vi "SEN_Loop.vi"() -> ()   [LabVIEW 2023, in "GameController_SEN.lvlib"]
uses:
  GameController_SEN.lvlib
  ENUM_SEN_State.ctl
  <vilib>/Rock Robotics/WPI/Joystick/WPI_JoystickDevRef.ctl
  <vilib>/Rock Robotics/WPI/Joystick/WPI_JoystickDeviceEnum.ctl
  ENUM_SEN_Action.ctl
  RoboRIO Utilities/Global_STOP.vi
  Global_SEN_Data Out.vi
panel:
  out "Input Bool Data":bool
  out "Output DBL Data":dbl
  out "Cycle Time (S)":dbl format="%.3g"
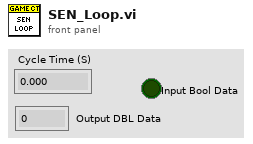
[diagram p1: front panel]
types:
  T1 = typedef "WPI_JoystickDevRef.ctl" = cluster{"Device":T2}
  T2 = typedef "WPI_JoystickDeviceEnum.ctl" = enum16{"USB 0", "USB 1", "USB 2", "USB 3", "USB 4", "USB 5"}
  T3 = typedef "GameController_SEN.lvlib/ENUM_SEN_State.ctl" = enum16{"Startup", "Enable", "Shutdown"}
  T4 = typedef "GameController_SEN.lvlib/ENUM_SEN_Action.ctl" = enum16{"No Action", "Reset Time", "Read Enable", "Read Disable"}
  T5 = cluster{"Sensor Ref 1":T1, "Sensor Ref 0":T1, "State":T3, "Previous State":T3, "Current Time":timestamp, "Previous Time":timestamp, "Start Time":timestamp, "Target Time (ms)":u32, "Cycle Time(S)":dbl, "SEN Input":bool, "SEN Output DBL":dbl, "Read Enable":bool, "Axes 0":dbl[], "Buttons 0":bool[], "POVs 0":i16[], "Axes 1":dbl[], "Buttons 1":bool[], "POVs 1":i16[]}
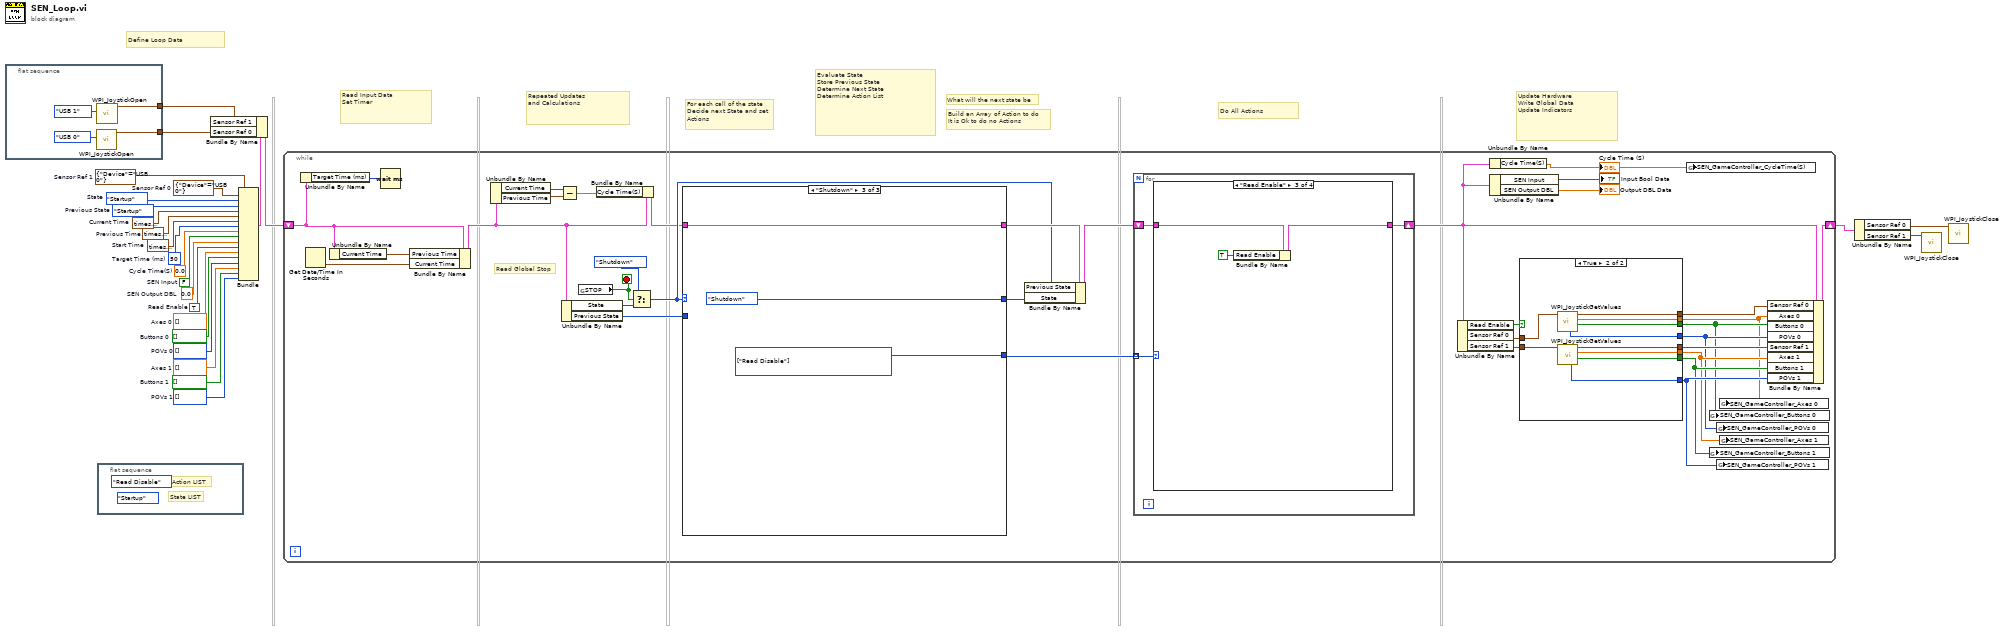
[diagram p0: block diagram]
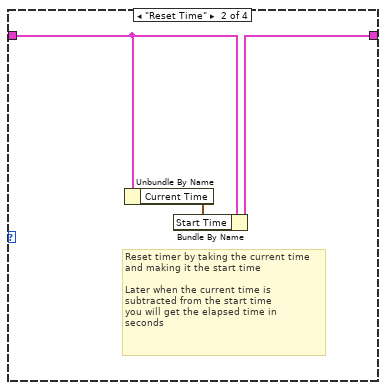
[diagram p4: hidden frame]
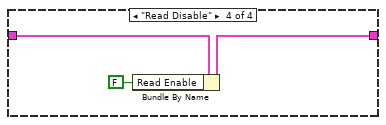
[diagram p5: hidden frame]
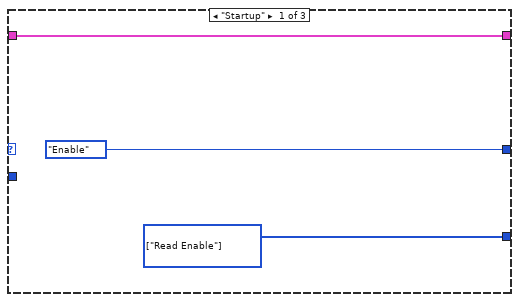
[diagram p6: hidden frame]
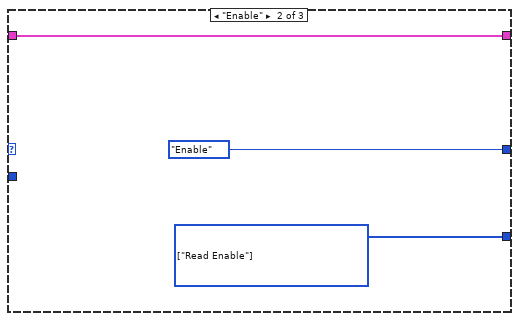
[diagram p7: hidden frame]
diagram:
  w1 = T1 {"Device"=enum."USB 0"}  # Sensor Ref 0
  w2 = T1 {"Device"=enum."USB 0"}  # Sensor Ref 1
  w5 = i16[] []  # POVs 1
  w6 = bool[] []  # Buttons 1
  w7 = dbl[] []  # Axes 1
  w8 = i16[] []  # POVs 0
  w9 = bool[] []  # Buttons 0
  w10 = dbl[] []  # Axes 0
  w15 = TRUE  # Read Enable
  w17 = 0.0  # Cycle Time(S)
  w18 = ENUM_SEN_State."Startup"  # Previous State
  w19 = timestamp(0 s since 1904-01-01)  # Previous Time
  w20 = u32 50  # Target Time (ms)
  w21 = 0.0  # SEN Output DBL
  w22 = FALSE  # SEN Input
  w23 = timestamp(0 s since 1904-01-01)  # Start Time
  w24 = timestamp(0 s since 1904-01-01)  # Current Time
  w25 = ENUM_SEN_State."Startup"  # State
  # "Build an Array of Action to do\nIt is Ok to do no Actions"
  # "What will the next state be"
  # "For each call of the state\nDecide next State and set\nActions"
  # "Define Loop Data"
  # "Repeated Updates\nand Calculations"
  # "Read Input Data\nSet Timer"
  # "Evaluate State\nStore Previous State\nDetermine Next State\nDetermine Action List"
  # "Do All Actions"
  # "Update Hardware\nWrite Global Data\nUpdate Indicators"
  n1 = flat-sequence {
    tunnel: [w28] -> w12
    tunnel: [w26] -> w11
    frame #0 {
      n2 = call <vilib>:"WPI_JoystickOpen.vi"("JoystickDevice"=WPI_JoystickDeviceEnum."USB 0") -> ("JoystickDevRef"=w28:T1)  [unwired: 10 in]
      n3 = call <vilib>:"WPI_JoystickOpen.vi"("JoystickDevice"=WPI_JoystickDeviceEnum."USB 1") -> ("JoystickDevRef"=w26:T1)  [unwired: 10 in]
    }
  }
  n4 = flat-sequence {
    frame #0 {
      (unwired) ENUM_SEN_State."Startup" ("State")
      (unwired) ENUM_SEN_Action."Read Disable" ("Action")
      # "State LIST"
      # "Action LIST"
    }
  }
  n5 = Bundle("Sensor Ref 1"=w2, "Sensor Ref 0"=w1, "State"=w25, "Previous State"=w18, "Current Time"=w24, "Previous Time"=w19, "Start Time"=w23, "Target Time (ms)"=w20, "Cycle Time(S)"=w17, "SEN Input"=w22, "SEN Output DBL"=w21, "Read Enable"=w15, "Axes 0"=w10, "Buttons 0"=w9, "POVs 0"=w8, "Axes 1"=w7, "Buttons 1"=w6, "POVs 1"=w5) -> (w14:T5)  [unwired: 1 in]
  n6 = Bundle By Name(cluster=w14, "Sensor Ref 1"=w11, "Sensor Ref 0"=w12) -> (w13:T5)
  n7 = while {
    shift-right: [w41] -> w16
    shift-left: w13 -> [w54]
    stop <- w59 stop-if-true
    # "Read Global Stop"
    n8 = Unbundle By Name(w54) -> ("Target Time (ms)"=w56:u32)
    n9 = Get Date/Time In Seconds() -> (seconds since 1Jan1904=w63:timestamp)
    n10 = Unbundle By Name(w54) -> ("Current Time"=w55:timestamp)
    n11 = Wait (ms)(milliseconds to wait=w56) -> ()  [unwired: 1 out]
    n12 = Bundle By Name(cluster=w54, "Previous Time"=w55, "Current Time"=w63) -> (w48:T5)
    n13 = Unbundle By Name(w48) -> ("Current Time"=w49:timestamp, "Previous Time"=w50:timestamp)
    n14 = Subtract(x=w49, y=w50) -> (x-y=w46:dbl)
    n15 = Unbundle By Name(w48) -> ("State"=w57:T3, "Previous State"=w53:T3)
    n16 = global read "Global_STOP.vi" "STOP"() -> (w59:bool)
    n17 = Bundle By Name(cluster=w48, "Cycle Time(S)"=w46) -> (w47:T5)
    n18 = Select(t=ENUM_SEN_State."Shutdown" ("State"), s=w59, f=w57) -> (s? t:f=w51:T3)
    n19 = case shown="\"Shutdown\"" w51 {
      tunnel: w47 -> [w91 w92 w97]
      tunnel: [w91 w92 w97] -> w61
      tunnel: [ENUM_SEN_State."Enable" ("State") ENUM_SEN_State."Enable" ("State") ENUM_SEN_State."Shutdown" ("State")] -> w60
      tunnel: [w90 w94 w95] -> w45
      tunnel: w53 -> [_ _ _]
      frame "Startup" {
        w90 = T4[] [enum."Read Enable"] items=["No Action", "Reset Time", "Read Enable", "Read Disable"] ("Actions")
      }
      frame "Enable" {
        w94 = T4[] [enum."Read Enable"] items=["No Action", "Reset Time", "Read Enable", "Read Disable"] ("Actions")
      }
      frame "Shutdown" {
        w95 = T4[] [enum."Read Disable"] items=["No Action", "Reset Time", "Read Enable", "Read Disable"] ("Actions")
      }
    }
    n20 = Bundle By Name(cluster=w61, "Previous State"=w51, "State"=w60) -> (w62:T5)
    n21 = for {
      tunnel: w45 -> [w78] mode=indexing
      shift-right: [w77] -> w42
      shift-left: w62 -> [w76]
      n22 = case shown="\"Read Enable\"" w78 {
        tunnel: w76 -> [w79 w82 w85 w88]
        tunnel: [w79 w81 w84 w87] -> w77
        frame "No Action" {
        }
        frame "Reset Time" {
          # "Reset timer by taking the current time\nand making it the start time\n\nLater when the current time is \nsubtracted from the start time\nyou will get the elapsed time in \nseconds"
          n23 = Unbundle By Name(w82) -> ("Current Time"=w80:timestamp)
          n24 = Bundle By Name(cluster=w82, "Start Time"=w80) -> (w81:T5)
        }
        frame "Read Enable" {
          n25 = Bundle By Name(cluster=w85, "Read Enable"=TRUE) -> (w84:T5)
        }
        frame "Read Disable" {
          n26 = Bundle By Name(cluster=w88, "Read Enable"=FALSE) -> (w87:T5)
        }
      }
    }
    n27 = Unbundle By Name(w42) -> ("Read Enable"=w39:bool, "Sensor Ref 0"=w43:T1, "Sensor Ref 1"=w38:T1)
    n28 = Unbundle By Name(w42) -> ("Cycle Time(S)"=w40:dbl)
    "Cycle Time (S)" <- w40
    n29 = Unbundle By Name(w42) -> ("SEN Input"=→"Input Bool Data":bool, "SEN Output DBL"=→"Output DBL Data":dbl)
    n30 = case shown="True" w39 {
      tunnel: w43 -> [w65 w75]
      tunnel: [w64 w72] -> w36
      tunnel: w38 -> [w64 w74]
      tunnel: [w65 w73] -> w37
      tunnel: [_ w71] -> w30
      tunnel: [_ w70] -> w31
      tunnel: [_ w69] -> w32
      tunnel: [_ w68] -> w33
      tunnel: [_ w67] -> w34
      tunnel: [_ w66] -> w35
      frame False {
      }
      frame True {
        n31 = call <vilib>:"WPI_JoystickGetValues.vi"("JoystickDevRef"=w75) -> ("Buttons"=w70:bool[], "Axes"=w71:dbl[], "JoystickDevRef"=w73:T1, "POVs"=w69:i16[])  [unwired: 6 in, 1 out]
        n32 = call <vilib>:"WPI_JoystickGetValues.vi"("JoystickDevRef"=w74) -> ("Buttons"=w67:bool[], "Axes"=w68:dbl[], "JoystickDevRef"=w72:T1, "POVs"=w66:i16[])  [unwired: 6 in, 1 out]
      }
    }
    n33 = global write "Global_SEN_Data Out.vi" "SEN_GameController_CycleTime(S)"(w40) -> ()
    n34 = global write "Global_SEN_Data Out.vi" "SEN_GameController_Buttons 0"(w31) -> ()
    n35 = global write "Global_SEN_Data Out.vi" "SEN_GameController_Buttons 1"(w34) -> ()
    n36 = global write "Global_SEN_Data Out.vi" "SEN_GameController_POVs 0"(w32) -> ()
    n37 = global write "Global_SEN_Data Out.vi" "SEN_GameController_POVs 1"(w35) -> ()
    n38 = global write "Global_SEN_Data Out.vi" "SEN_GameController_Axes 0"(w30) -> ()
    n39 = global write "Global_SEN_Data Out.vi" "SEN_GameController_Axes 1"(w33) -> ()
    n40 = Bundle By Name(cluster=w42, "Sensor Ref 0"=w37, "Axes 0"=w30, "Buttons 0"=w31, "POVs 0"=w32, "Sensor Ref 1"=w36, "Axes 1"=w33, "Buttons 1"=w34, "POVs 1"=w35) -> (w41:T5)
  }
  n41 = Unbundle By Name(w16) -> ("Sensor Ref 0"=w4:T1, "Sensor Ref 1"=w3:T1)
  n42 = call <vilib>:"WPI_JoystickClose.vi"("JoystickDevRef"=w3) -> ()  [unwired: 11 in]
  n43 = call <vilib>:"WPI_JoystickClose.vi"("JoystickDevRef"=w4) -> ()  [unwired: 11 in]
